vi "PH_Beckhoff_PP_PU.declare digital PSU OutputTags.vi"(3 "PUs":T1[](array[typedef])=[enum."MA-PU-1", enum."MA-PU-2"]) -> (0 "inverted?":bool[](array[boolean]), 1 "Tagnames":string[](array[string]))   [LabVIEW 2014, in "PH_Beckhoff_PP_PU.lvlib"]
uses:
  PH_Beckhoff_PP_PU.lvlib
  PH_Basics/PH_PP_Common/PH_PP_Common.PUs.ctl
  PH_Basics/PH_PP_Common/PH_PP_Common.PSU Tags.ctl
  PH_Basics/PH_PP_Common/PH_PP_Common.PSU Type.ctl
  PH_Basics/PH_PP_Common/PH_PP_Common.lvlib
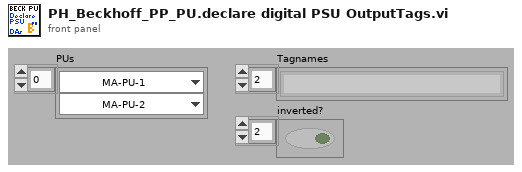
[diagram p1: front panel]
types:
  T1 = typedef "PH_PP_Common.lvlib/PH_PP_Common.PUs.ctl" = enum16{"no Info", "PA-19mm-1", "PA-19mm-2", "PA-45mm-PILC", "PA-45mm-MAIN", "MA-PU-1", "MA-PU-2", "MA-PU-3", "MA-PU-4", "MA-PU-5", "MA-PU-6", "MA-FR", "MA-PILC", "PA-45mm-DP"}
  T2 = typedef "PH_PP_Common.lvlib/PH_PP_Common.PSU Tags.ctl" = enum16{"voltage-indicator", "peak-detect", "current", "voltage", "inihibit-indicator", "end-of-charge", "HV-on-indicator", "overtemperature", "interlock-indicator", "load-fault", "sum-fault", "HV-off-indicator", "DC-ok", "inhibit", "HV-on", "interlock", "reset", "Status", "Limits"}
  T3 = typedef "PH_PP_Common.lvlib/PH_PP_Common.PSU Type.ctl" = enum16{"none", "Maxwell Standard", "DEL", "Maxwell ALE", "Continuum 601k"}
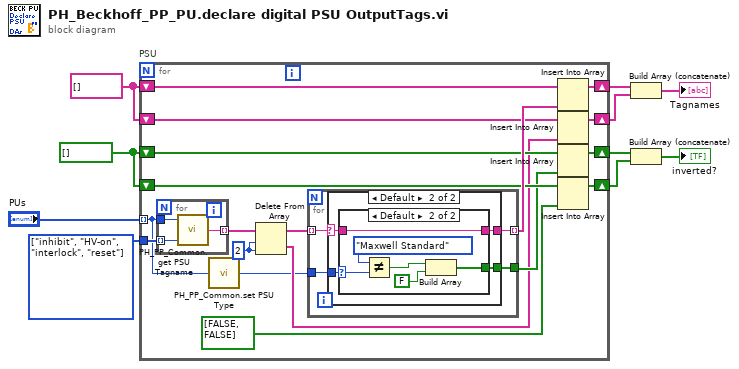
[diagram p0: block diagram]
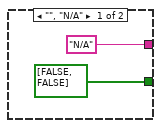
[diagram p2: hidden frame]
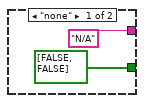
[diagram p3: hidden frame]
diagram:
  w2 = T2[] [enum."inhibit", enum."HV-on", enum."interlock", enum."reset"] items=["voltage-indicator", "peak-detect", "current", "voltage", "inihibit-indicator", "end-of-charge", "HV-on-indicator", "overtemperature", "interlock-indicator", "load-fault", "sum-fault", "HV-off-indicator", "DC-ok", "inhibit", "HV-on", "interlock", "reset", "Status", "Limits"]
  w9 = bool[] []
  w10 = string[] []
  n1 = for "PSU" {
    shift-right: [w27] -> w7
    shift-left: w10 -> [w26]
    shift-right: [w25] -> w8
    shift-left: w9 -> [w24]
    shift-right: [w23] -> w5
    shift-left: w10 -> [w22]
    shift-right: [w21] -> w3
    shift-left: w9 -> [w20]
    tunnel: "PUs" -> [w11] mode=indexing
    tunnel: w2 -> [w17]
    w15 = 2 ("length")
    n2 = for "PSU" {
      tunnel: w11 -> [w31]
      tunnel: w17 -> [w30] mode=indexing
      tunnel: [w29] -> w16 mode=indexing
      n3 = call "PH_PP_Common.get PSU Tagname.vi"("PSU Tag"=w30, "PU"=w31) -> ("PSU Tagname"=w29:string)  [unwired: 1 in]
    }
    n4 = call "PH_PP_Common.set PSU Type.vi"("PU"=w11) -> ("PSU Type"=w12:T3)
    n5 = Delete From Array(array=w16, length=w15, index=w15) -> (deleted portion=w13:string[], array with subset deleted=w14:string[])
    n6 = for {
      tunnel: w12 -> [w35]
      tunnel: [w34] -> w28 mode=indexing
      tunnel: [w33] -> w18
      tunnel: w14 -> [w32] mode=indexing
      n7 = case shown="Default" w32 {
        selector: w32 -> [_ w38]
        tunnel: w35 -> [_ w41]
        tunnel: ["N/A" w40] -> w34
        tunnel: [bool[] [FALSE, FALSE] w39] -> w33
        frame "", "N/A" {
        }
        frame Default {
          n8 = case shown="Default" w41 {
            selector: w41 -> [_ w48]
            tunnel: ["N/A" w49] -> w40
            tunnel: [bool[] [FALSE, FALSE] w45] -> w39
            tunnel: w38 -> [_ w49]
            frame "none" {
            }
            frame Default {
              n9 = Not Equal?(x=PH_PP_Common.PSU_Type."Maxwell Standard" ("PSU 2 Type"), y=w48) -> (x != y?=w46:bool)
              n10 = Build Array(w46, FALSE ("element")) -> (w45:bool[])
            }
          }
        }
      }
    }
    n11 = Insert Into Array(array=w26, new element=w28) -> (w27:string[])  [unwired: 1 in]
    n12 = Insert Into Array(array=w22, new element=w13) -> (w23:string[])  [unwired: 1 in]
    n13 = Insert Into Array(array=w24, new element=w18) -> (w25:bool[])  [unwired: 1 in]
    n14 = Insert Into Array(array=w20, new element=bool[] [FALSE, FALSE]) -> (w21:bool[])  [unwired: 1 in]
  }
  n15 = Build Array (concatenate)(w7, w5) -> (→"Tagnames":string[])
  n16 = Build Array (concatenate)(w8, w3) -> (→"inverted?":bool[])
